vi "Connect to Server.vi"(4 "timeout (2000 ms)":i32=2000, 5 "Connect Flags":T3={"Reserved"=FALSE, "Clean Session"=TRUE, "Will Flag"=FALSE, "Will QoS 1"=FALSE, "Will QoS 2"=FALSE, "Will Retain"=FALSE, "Password Flag"=FALSE, "User Name Flag"=FALSE}, 6 "Keep Alive (s)":u16, 7 "Payload":T2, 8 "error in (no error)":errorcluster, 11 "Client in":refnum<class "Client.lvclass">) -> (0 "error out":errorcluster, 1 "timed out":bool, 2 "Return Code":T1=enum."Server Unavailable", 3 "Client out":refnum<class "Client.lvclass">)   [LabVIEW 2013, in "MQTT Client.lvlib" / "Client.lvclass"]
uses:
  Client.lvclass
  <vilib>/LabVIEW Open Source Project/MQTT Control Packets/Control Packets/CONNECT/ConnectFlags -- cluster.ctl
  <vilib>/LabVIEW Open Source Project/MQTT Control Packets/Control Packets/CONNACK/Connect Return Code -- enum.ctl
  <vilib>/LabVIEW Open Source Project/MQTT Control Packets/Control Packets/CONNACK/CONNACK.lvclass
  <vilib>/LabVIEW Open Source Project/MQTT Connection/MQTT_Base/Base Class/MQTT_Base.lvclass/MQTT_Base.ctl
  Client.lvclass/Client.ctl
  <vilib>/LabVIEW Open Source Project/MQTT Control Packets/Control Packets/ControlPacket/ControlPacket.lvclass
  <vilib>/LabVIEW Open Source Project/MQTT Control Packets/Control Packets/CONNECT/CONNECT.lvclass
  <vilib>/LabVIEW Open Source Project/MQTT Connection/MQTT_Base/Session/Session.lvclass
  <vilib>/LabVIEW Open Source Project/MQTT Connection/MQTT_Base/Base Class/MQTT_Base.lvclass
  Session.Client/Session.Client.lvclass
  <vilib>/LabVIEW Open Source Project/MQTT Connection/MQTT_Connection/Connection/Connection.lvclass
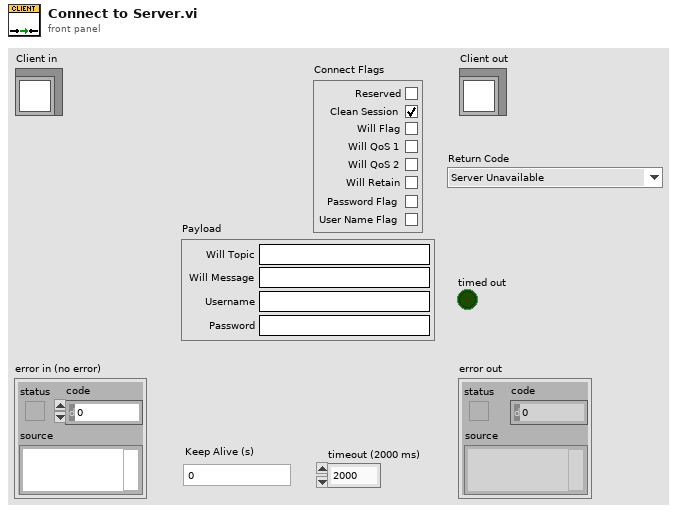
[diagram p1: front panel]
types:
  T1 = typedef "MQTT_Control_Packets.lvlib/CONNACK.lvclass/Connect Return Code -- enum.ctl" = enum16{"Connection accepted", "Unacceptable protocol version", "Identifier Rejected", "Server Unavailable", "Bad Username or Password", "Not Authorized"}
  T2 = cluster{"Will Topic":string, "Will Message":string, "Username":string, "Password":string}
  T3 = typedef "MQTT_Control_Packets.lvlib/CONNECT.lvclass/ConnectFlags -- cluster.ctl" = cluster{"Reserved":bool, "Clean Session":bool, "Will Flag":bool, "Will QoS 1":bool, "Will QoS 2":bool, "Will Retain":bool, "Password Flag":bool, "User Name Flag":bool}
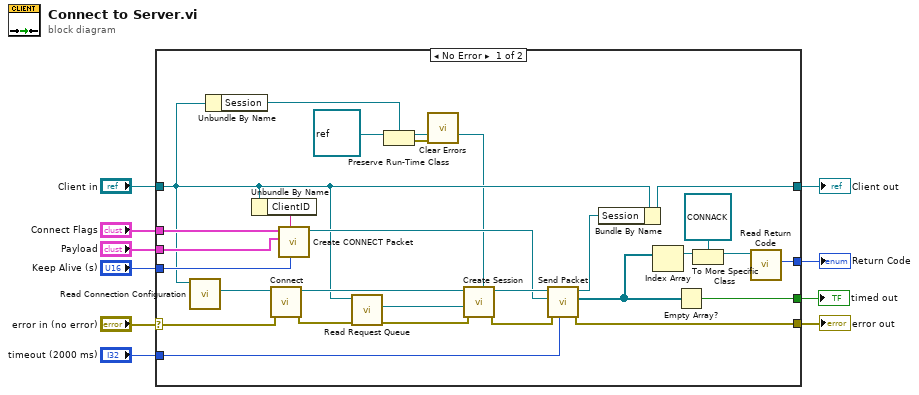
[diagram p0: block diagram]
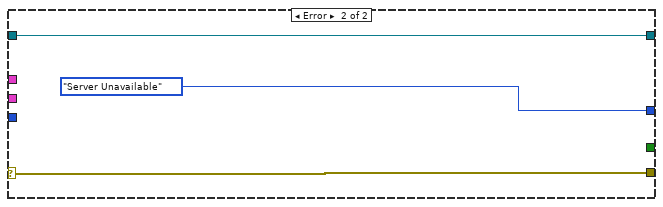
[diagram p2: hidden frame]
diagram:
  n1 = case shown="No Error" "error in (no error)" {
    selector: "error in (no error)" -> [w19 w41]
    tunnel: [w21 w41] -> w9
    tunnel: [w38 w40] -> w7
    tunnel: "Client in" -> [w15 w40]
    tunnel: "Connect Flags" -> [w37 _]
    tunnel: "Payload" -> [w36 _]
    tunnel: "Keep Alive (s)" -> [w35 _]
    tunnel: [w24 _] -> w3
    tunnel: "timeout (2000 ms)" -> [w30 _]
    tunnel: [w26 Connect_Return_Code_--_enum."Server Unavailable" ("Return Code")] -> w1
    frame No Error {
      n2 = call <vilib>:"Read Connection Configuration.vi"("MQTT_Base in"=w15) -> ("Connection Configuration"=w16:refnum<class "Connection.lvclass">)  [unwired: 8 in, 2 out]
      n3 = Unbundle By Name(w15) -> ("Session"=w14:refnum<class "Session.Client.lvclass">)
      n4 = Unbundle By Name(w15) -> ("ClientID"=w34:string)
      n5 = call <vilib>:"Connect.vi"("error in (no error)"=w19, "Connection in"=w16) -> ("error out"=w18:errorcluster, "Connection out"=w17:refnum<class "Connection.lvclass">)  [unwired: 8 in]
      n6 = call <vilib>:"Create CONNECT Packet.vi"("Keep Alive (s)"=w35, "Client ID (empty: generate new)"=w34, "Payload"=w36, "Connect Flags"=w37) -> ("CONNECT"=w31:refnum<class "CONNECT.lvclass">)  [unwired: 5 in, 2 out]
      n7 = call <vilib>:"Read Request Queue.vi"("error in (no error)"=w18, "MQTT_Base in"=w15) -> ("error out"=w23:errorcluster, "Request"=w33:refnum<queue>)  [unwired: 7 in, 1 out]
      n8 = Preserve Run-Time Class(object in=refnum<class> refnum ("LabVIEW Object"), 2:w14) -> (object out=w11:refnum<class "Session.Client.lvclass">, error out=w12:errorcluster)  [unwired: 1 in]
      n9 = call <vilib>:"Clear Errors.vi"("error in (no error)"=w12) -> ()  [unwired: 6 in, 1 out]
      n10 = call <vilib>:"Create Session.vi"("Session in"=w11, "error in (no error)"=w23, "Request"=w33, "Connection"=w17) -> ("error out"=w20:errorcluster, "Session"=w32:refnum<class "Session.Client.lvclass">)  [unwired: 6 in]
      n11 = call "Send Packet.vi"("timeout (0ms : no ack)"=w30, "error in (no error)"=w20, "Packet"=w31, "Session"=w32) -> ("error out"=w21:errorcluster, "Response"=w25:refnum<class "ControlPacket.lvclass">[], "Session"=w22:refnum<class "Session.Client.lvclass">)  [unwired: 4 in, 1 out]
      n12 = Bundle By Name(cluster=w15, "Session"=w22) -> (w38:refnum<class "Client.lvclass">)
      n13 = Index Array(array=w25) -> (element=w29:refnum<class "ControlPacket.lvclass">)  [unwired: 1 in]
      n14 = Empty Array?(array=w25) -> (empty?=w24:bool)
      n15 = To More Specific Class(target class=refnum<class "CONNACK.lvclass"> refnum ("CONNACK.lvclass"), reference=w29) -> (specific class reference=w27:refnum<class "CONNACK.lvclass">)  [unwired: 1 in, 1 out]
      n16 = call <vilib>:"Read Return Code.vi"("CONNACK in"=w27) -> ("Return Code"=w26:T1)  [unwired: 8 in, 2 out]
    }
    frame Error {
    }
  }
  "error out" <- w9
  "Client out" <- w7
  "timed out" <- w3
  "Return Code" <- w1
